vi "Get Object By ID.vi"(8 "error in (no error)":errorcluster, 10 "ID":string, 11 "Editor.lvclass in":refnum<data-value>) -> (0 "error out":errorcluster, 2 "SerializableObject out":refnum<class "SerializableObject.lvclass">, 3 "Editor.lvclass out":refnum<data-value>)   [LabVIEW 2015, in "Editor.lvclass"]
uses:
  Editor.lvclass
  SerializableObject/SerializableObject.lvclass
  Project.lvclass
  Step.lvclass
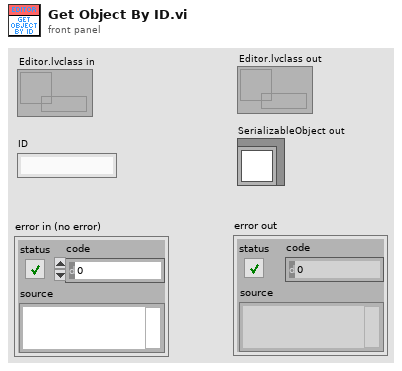
[diagram p1: front panel]
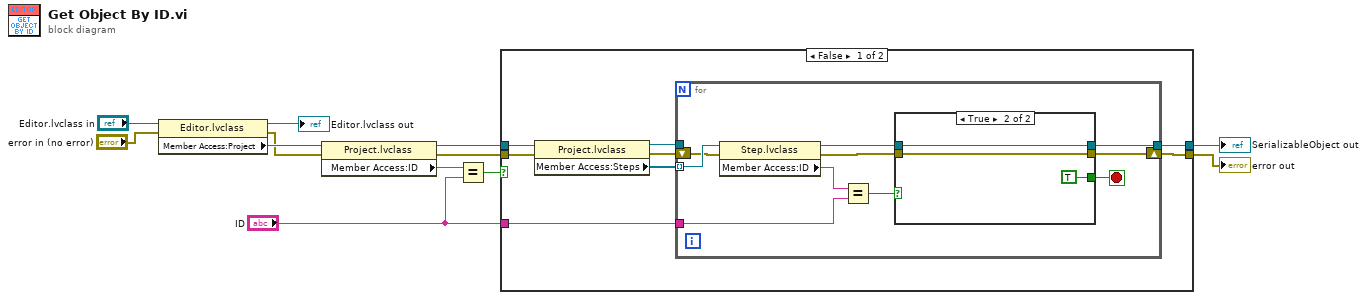
[diagram p0: block diagram]
diagram:
  n1 = property class="Editor.lvclass"(reference="Editor.lvclass in", error in="error in (no error)") -> (reference out=→"Editor.lvclass out":refnum<data-value>, error out=w2:errorcluster, "Member Access:Project"=w3:refnum<class "Project.lvclass">)
  n2 = property class="Project.lvclass"(reference=w3, error in=w2) -> (reference out=w10:refnum<class "Project.lvclass">, error out=w9:errorcluster, "Member Access:ID"=w12:string)
  n3 = Equal?(x=w12, y="ID") -> (x = y?=w11:bool)
  n4 = case shown="False" w11 {
    tunnel: w10 -> [w20 w35]
    tunnel: w9 -> [w19 w34]
    tunnel: "ID" -> [w15 _]
    tunnel: [w14 w35] -> w6
    tunnel: [w13 w34] -> w7
    frame False {
      n5 = property class="Project.lvclass"(reference=w20, error in=w19) -> (reference out=w18:refnum<class "Project.lvclass">, error out=w17:errorcluster, "Member Access:Steps"=w16:refnum<class "Step.lvclass">[])
      n6 = for {
        tunnel: w18 -> [_]
        shift-right: [w23] -> w13
        shift-left: w17 -> [w27]
        tunnel: w16 -> [w30] mode=indexing
        tunnel: w15 -> [w28]
        tunnel: [w22] -> w14
        stop <- w21 stop-if-true
        n7 = property class="Step.lvclass"(reference=w30, error in=w27) -> (reference out=w26:refnum<class "Step.lvclass">, error out=w25:errorcluster, "Member Access:ID"=w29:string)
        n8 = Equal?(x=w29, y=w28) -> (x = y?=w24:bool)
        n9 = case shown="True" w24 {
          tunnel: w26 -> [_ w32]
          tunnel: w25 -> [_ w33]
          tunnel: [_ w33] -> w23
          tunnel: [_ w32] -> w22
          tunnel: [_ TRUE] -> w21
          frame False {
          }
          frame True {
          }
        }
      }
    }
    frame True {
    }
  }
  "error out" <- w7
  "SerializableObject out" <- w6
